vi "CLosed Loop Gain Tool .vi"() -> ()   [LabVIEW 2018]
uses:
  <vilib>/DAQmx/write.llb/DAQmx Write (Analog DBL 1Chan 1Samp).vi
  <vilib>/DAQmx/read.llb/DAQmx Read (Analog DBL 1Chan 1Samp).vi
  <vilib>/DAQmx/create/channels.llb/DAQmx Create Channel (AI-Voltage-Basic).vi
  <vilib>/DAQmx/miscellaneous.llb/DAQmx Fill In Error Info.vi
  <vilib>/addons/control/pid/pid.llb/PID Gain Schedule (DBL).vi
  <vilib>/addons/control/pid/autopid.llb/PID Online Autotuning (Step Closed Loop).vi
  <vilib>/addons/control/pid/pid.llb/PID Advanced (DBL).vi
  <vilib>/addons/control/pid/NI_PID_pid.lvlib
  <vilib>/ptbypt/NI_PtbyPt.lvlib
  <vilib>/addons/control/pid/NI_PID_autopid.lvlib
panel:
  out "Scaled MV":dbl(slide) scale=0.0..2000.0
  in  "Target Pressure(in Torr)":dbl
  out "Pressure Readout  (in Torr)":dbl(slide) scale=0.0..1000.0
  out "Pressure (in torr)":dbl
  in  "Sampling Time dt (s)":dbl=0.05 min=0.001 step=0.01 format="%#.3p"
  in  "Stop":bool
  out "SP and PV":cluster{"initial PV":dbl, "SP1:":dbl}(graph)={"initial PV"=50.98160323470328, "SP1:"=50.98039215686275}
  out "PID Gains":T1={"proportional gain (Kc)"=6.925505792902687, "integral time (Ti, min)"=0.004930412653813362, "derivative time (Td, min)"=0.0} {"derivative time (Td, min)" format="%#.6g"; "integral time (Ti, min)" format="%#.6g"; "proportional gain (Kc)" format="%#.6g"}
  in  "Autotune":bool
  in  "Replace gains":bool
  out "MV":dbl(graph)
  out "tuned PID gains":T1={"proportional gain (Kc)"=1.9838195929127882, "integral time (Ti, min)"=0.01995856284686879, "derivative time (Td, min)"=0.0} {"derivative time (Td, min)" format="%#.6g"; "integral time (Ti, min)" format="%#.6g"; "proportional gain (Kc)" format="%#.6g"}
  in  "autotuning parameters":T2={"Type of Controller"=2, "relay cycles"=3, "amplitude"=1.0, "control specifications"=2, "PV noise level"=0.1} {"PV noise level" format="%.2f"; "control specifications" items=["fast", "normal", "slow"]; "amplitude" format="%.2f"; "Type of Controller" items=["P", "PI", "PID"]}
  in  "Reinitialize":bool
  in  "Automatic":bool=TRUE
  in  "alpha":dbl=nan format="%.2f"
  in  "PID gain schedule":T3(array[cluster])=[{"PID gains"={"Kc"=7.0, "Ti"=0.001, "Td"=0.0}, "max value"=0.0}] {"max value" format="%.2f"; "PID gains"."Td" format="%#.3g"; "PID gains"."Ti" format="%#.3g"; "PID gains"."Kc" format="%#.3g"}
  in  "Insert gains":bool
  out "Gain Scheduling":i32
  # "Gain Scheduling"
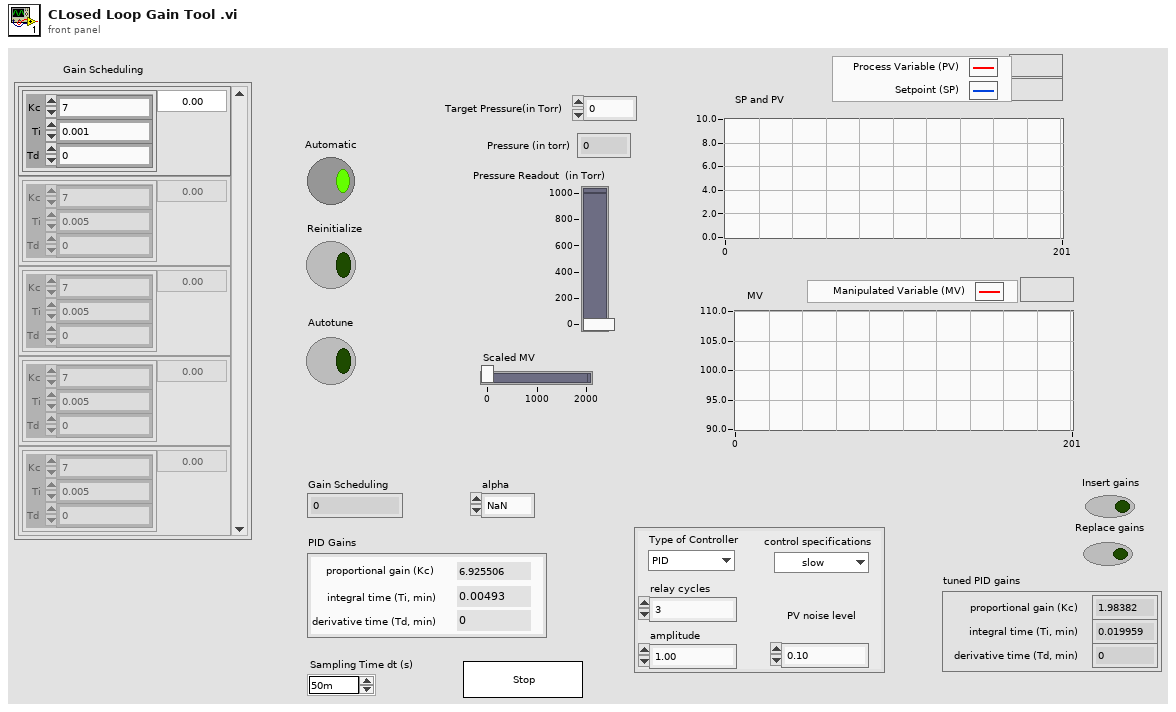
[diagram p1: front panel]
types:
  T1 = cluster{"proportional gain (Kc)":dbl, "integral time (Ti, min)":dbl, "derivative time (Td, min)":dbl}
  T2 = cluster{"Type of Controller":u16, "relay cycles":i32, "amplitude":dbl, "control specifications":u16, "PV noise level":dbl}
  T3 = cluster{"PID gains":cluster{"Kc":dbl, "Ti":dbl, "Td":dbl}, "max value":dbl}[]
  T4 = cluster{"tuned PID gains":cluster{"proportional gain (Kc)":dbl, "integral time (Ti, min)":dbl, "derivative time (Td, min)":dbl}, "Target Pressure(in Torr)":dbl}
  T5 = cluster{"PID gains":cluster{"Kc":dbl, "Ti":dbl, "Td":dbl}, "max value":dbl}
  T6 = cluster{"tuned PID gains":cluster{"proportional gain (Kc)":dbl, "integral time (Ti, min)":dbl, "derivative time (Td, min)":dbl}, "max value":dbl}
  T7 = cluster{"Pressure Readout  (in Torr)":dbl, "Target Pressure(in Torr)":dbl}
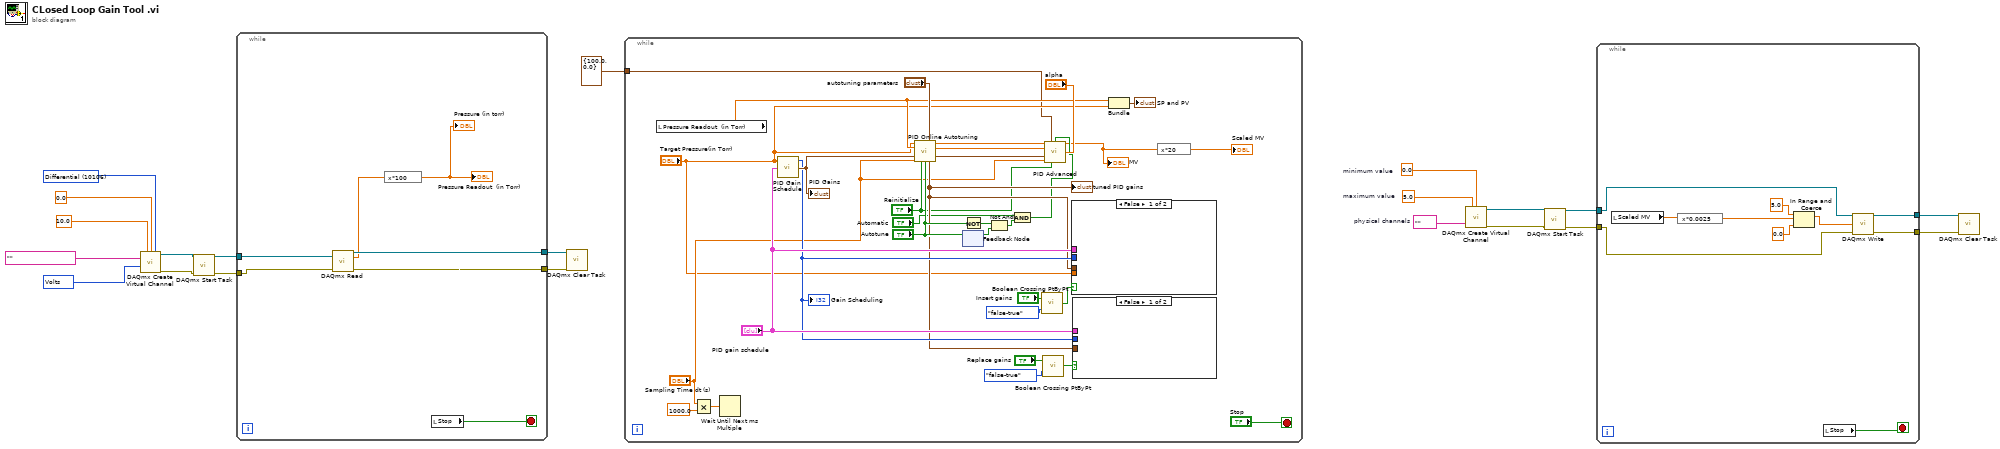
[diagram p0: block diagram]
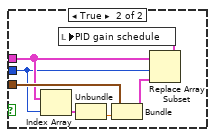
[diagram p2: hidden frame]
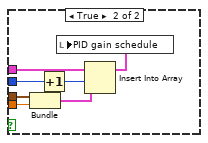
[diagram p3: hidden frame]
diagram:
  w4 = tag ""  # physical channels
  w5 = 0.0  # minimum value
  w6 = 5.0  # maximum value
  w11 = 10348 items=["Volts"=10348, "From Custom Scale"=10065] ("units")
  w13 = 10106 items=["Default"=-1, "RSE"=10083, "NRSE"=10078, "Differential"=10106, "Pseudodifferential"=12529] ("input terminal configuration")
  n1 = call-poly <vilib>:"DAQmx Create Virtual Channel.vi"("maximum value"=10.0, "minimum value"=0.0, "input terminal configuration"=w13, "physical channels"=tag "", "units"=w11) -> ("task out"=w21:refnum<k21>, "error out"=w20:errorcluster)  [unwired: 9 in]
  n2 = call <vilib>:"DAQmx Start Task.vi"("task/channels in"=w21, "error in"=w20) -> ("task out"=w19:refnum<k21>, "error out"=w17:errorcluster)  [unwired: 12 in]
  n3 = while {
    tunnel: w19 -> [w28]
    tunnel: [w27] -> w18
    tunnel: w17 -> [w26]
    tunnel: [w25] -> w16
    stop <- w22 stop-if-true
    n4 = call-poly <vilib>:"DAQmx Read.vi"("task/channels in"=w28, "error in"=w26) -> ("task out"=w27:refnum<k21>, "data"=w24:dbl, "error out"=w25:errorcluster)  [unwired: 11 in]
    n5 = expression code="x*100"(w24) -> (→"Pressure Readout  (in Torr)" →"Pressure (in torr)":dbl)
    n6 = local read "Stop"() -> (w22:bool)
  }
  n7 = call <vilib>:"DAQmx Clear Task.vi"("task in"=w18, "error in"=w16) -> ()  [unwired: 13 in, 1 out]
  n8 = while {
    tunnel: cluster{"output high":dbl, "output low":dbl} {"output high"=100.0, "output low"=0.0} ("output range") -> [w29]
    stop <- "Stop" stop-if-true
    n9 = local read "Pressure Readout  (in Torr)"() -> (w37:dbl)
    n10 = Multiply(x="Sampling Time dt (s)", y=1000.0) -> (x*y=w35:dbl)
    n11 = Wait Until Next ms Multiple(millisecond multiple=w35) -> ()  [unwired: 1 out]
    n12 = call-poly <vilib>:"PID Gain Schedule.vi"("PID gain schedule"="PID gain schedule", "gain scheduling value"="Target Pressure(in Torr)") -> ("PID gains out"=w49:T1, "index out"=w44:i32)  [unwired: 2 in]
    "PID Gains" <- w49
    "Gain Scheduling" <- w44
    n13 = call-poly <vilib>:"PID Online Autotuning.vi"("setpoint"="Target Pressure(in Torr)", "autotuning parameters"="autotuning parameters", "process variable"=w37, "PID gains in"=w49, "dt (s)"="Sampling Time dt (s)", "reinitialize? (F)"="Reinitialize", "autotune? (F)"="Autotune") -> ("setpoint out"=w59:dbl, "process variable out"=w58:dbl, "PID gains out"=w56:T1, "tuned PID gains"=w43:T1)  [unwired: 4 in, 1 out]
    "tuned PID gains" <- w43
    n14 = feedback #1() -> (w55:bool)  [unwired: 1 in]
    n15 = feedback-in #1("Autotune") -> ()
    n16 = Not(x="Autotune") -> (.not. x?=w52:bool)
    n17 = Not And(1:w55, 2:w52) -> (0:w53:bool)
    n18 = And(x="Automatic", y=w53) -> (x .and. y?=w40:bool)
    n19 = call <vilib>:"Boolean Crossing PtByPt.vi"("direction"=enum16{"either", "false-true", "true-false"}."false-true", "input"="Insert gains") -> ("crossing"=w50:bool)  [unwired: 1 in]
    n20 = call <vilib>:"Boolean Crossing PtByPt.vi"("direction"=enum16{"either", "false-true", "true-false"}."false-true", "input"="Replace gains") -> ("crossing"=w46:bool)  [unwired: 1 in]
    n21 = call-poly <vilib>:"PID Advanced.vi"("setpoint"=w59, "output range"=w29, "auto? (T)"=w40, "process variable"=w58, "alpha"="alpha", "PID gains"=w56, "dt (s)"="Sampling Time dt (s)", "reinitialize? (F)"="Reinitialize") -> ("output"=w31:dbl)  [unwired: 6 in, 1 out]
    "MV" <- w31
    n22 = case shown="False" w50 {
      tunnel: w43 -> [_ w74]
      tunnel: "Target Pressure(in Torr)" -> [_ w73]
      tunnel: "PID gain schedule" -> [_ w71]
      tunnel: w44 -> [_ w69]
      frame False {
      }
      frame True {
        n23 = Bundle("tuned PID gains"=w74, "Target Pressure(in Torr)"=w73) -> (w72:T4)  [unwired: 1 in]
        n24 = Increment(x=w69) -> (x+1=w68:i32)
        n25 = Insert Into Array(array=w71, index=w68, new element=w72) -> (w70:T3)
        n26 = local write "PID gain schedule"(w70) -> ()
      }
    }
    n27 = case shown="False" w46 {
      tunnel: w43 -> [_ w67]
      tunnel: "PID gain schedule" -> [_ w64]
      tunnel: w44 -> [_ w63]
      frame False {
      }
      frame True {
        n28 = Index Array(array=w64, index=w63) -> (element=w62:T5)
        n29 = Unbundle(w62) -> ("max value"=w61:dbl)  [unwired: 1 out]
        n30 = Bundle("tuned PID gains"=w67, "max value"=w61) -> (w65:T6)  [unwired: 1 in]
        n31 = Replace Array Subset(array=w64, new element=w65, index=w63) -> (w66:T3)
        n32 = local write "PID gain schedule"(w66) -> ()
      }
    }
    n33 = Bundle("Pressure Readout  (in Torr)"=w37, "Target Pressure(in Torr)"="Target Pressure(in Torr)") -> (→"SP and PV":T7)  [unwired: 1 in]
    n34 = expression code="x*20"(w31) -> (→"Scaled MV":dbl)
  }
  n35 = call-poly <vilib>:"DAQmx Create Virtual Channel.vi"("maximum value"=w6, "minimum value"=w5, "physical channels"=w4) -> ("task out"=w8:refnum<k21>, "error out"=w7:errorcluster)  [unwired: 11 in]
  n36 = call <vilib>:"DAQmx Start Task.vi"("task/channels in"=w8, "error in"=w7) -> ("task out"=w3:refnum<k21>, "error out"=w2:errorcluster)  [unwired: 12 in]
  n37 = while {
    tunnel: [w84] -> w10
    tunnel: [w83] -> w9
    tunnel: w3 -> [w78]
    tunnel: w2 -> [w77]
    stop <- w75 stop-if-true
    n38 = local read "Scaled MV"() -> (w76:dbl)
    n39 = expression code="x*0.0025"(w76) -> (w81:dbl)
    n40 = In Range and Coerce(upper limit=5.0, x=w81, lower limit=0.0) -> (coerced(x)=w82:dbl)  [unwired: 1 out]
    n41 = local read "Stop"() -> (w75:bool)
    n42 = call-poly <vilib>:"DAQmx Write.vi"("task/channels in"=w78, "data"=w82, "error in"=w77) -> ("task out"=w84:refnum<k21>, "error out"=w83:errorcluster)  [unwired: 10 in, 1 out]
  }
  n43 = call <vilib>:"DAQmx Clear Task.vi"("task in"=w10, "error in"=w9) -> ()  [unwired: 13 in, 1 out]
